vi "SVPO Integration (1 CH DBL WDT) with IC.vi"(6 "reset filters":bool, 7 "desired base units for length":i32(ring)=-1 items=["no change"=-1, "m"=0, "mm"=2, "microns"=3, "in"=1, "mils"=5], 8 "initial conditions":T1 {"filter state"."initial highpass filter state" format="%.2f"; "filter state"."initial integration fiter state"."y(n-2) state" format="%.2f"; "filter state"."initial integration fiter state"."x(n-2) state" format="%.2f"; "filter state"."initial integration fiter state"."y(n-1) state" format="%.2f"; "filter state"."initial integration fiter state"."x(n-1) state" format="%.2f"; "filter coefficents"."highpass filter coefficients"."Forward Coefficients" format="%.2f"; "filter coefficents"."highpass filter coefficients"."Reverse Coefficients" format="%.2f"; "filter coefficents"."integration filter coefficients"."alpha" format="%.2f"; "filter coefficents"."integration filter coefficients"."gamma" format="%.2f"; "filter coefficents"."integration filter coefficients"."beta" format="%.2f"}, 9 "highpass cutoff frequency [Hz]":dbl=1.0 format="%.2f", 11 "scaled signal [EU]":waveform(dbl)) -> (0 "final conditions":T1 {"filter state"."initial highpass filter state" format="%.2f"; "filter state"."initial integration fiter state"."y(n-2) state" format="%.2f"; "filter state"."initial integration fiter state"."x(n-2) state" format="%.2f"; "filter state"."initial integration fiter state"."y(n-1) state" format="%.2f"; "filter state"."initial integration fiter state"."x(n-1) state" format="%.2f"; "filter coefficents"."highpass filter coefficients"."Forward Coefficients" format="%.2f"; "filter coefficents"."highpass filter coefficients"."Reverse Coefficients" format="%.2f"; "filter coefficents"."integration filter coefficients"."alpha" format="%.2f"; "filter coefficents"."integration filter coefficients"."gamma" format="%.2f"; "filter coefficents"."integration filter coefficients"."beta" format="%.2f"}, 3 "integrated signal [EU*s]":waveform(dbl))   [LabVIEW 2017, in "SoundVib_Integration.lvlib"]
doc: "Converts acceleration to velocity or velocity to displacement using a time-domain waveform as the input. Wire data to the <B>scaled signal [EU]</B> input to determine the polymorphic instance to use or manually select the instance. This VI performs Single Integration only. You can pass the integrated signal [EU*s] output to the scaled signal [EU] input of second call to this VI to perform double integration."
uses:
  <vilib>/addons/Sound and Vibration/svt_Integration/SoundVib_Integration.lvlib
  <vilib>/addons/_NISVFA/_Shared subVIs/Controls/svc_Integration State.ctl
  <vilib>/addons/Sound and Vibration/svt_Integration/subVIs/svl_Apply Highpass Filter with IC.vi
  <vilib>/addons/Sound and Vibration/svt_Integration/subVIs/svl_Low Pass [Order 1] No State.vi
  <vilib>/addons/Sound and Vibration/svt_Integration/subVIs/svl_Design HighPass Filter.vi
  <vilib>/addons/Sound and Vibration/svt_Integration/subVIs/svl_RC Filter Coefficients.vi
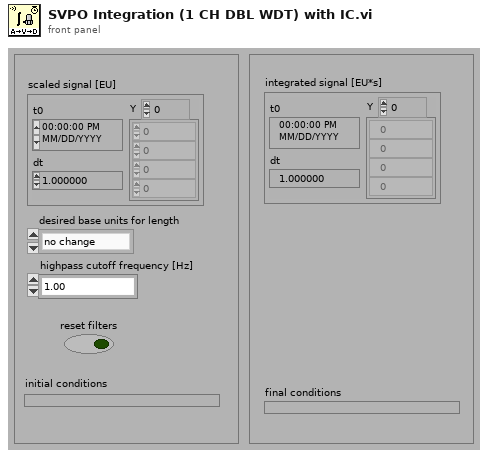
[diagram p1: front panel]
types:
  T1 = typedef "svc_Integration State.ctl" = cluster{"filter coefficents":cluster{"integration filter coefficients":cluster{"beta":dbl, "gamma":dbl, "alpha":dbl}, "highpass filter coefficients":cluster{"filter structure":enum32{"IIR 2nd Order", "IIR 4th Order"}, "Reverse Coefficients":dbl[], "Forward Coefficients":dbl[]}}, "filter state":cluster{"initial integration fiter state":cluster{"x(n-1) state":dbl, "y(n-1) state":dbl, "x(n-2) state":dbl, "y(n-2) state":dbl}, "initial highpass filter state":dbl[]}}
  T2 = enum16{"single integration", "double integration"}
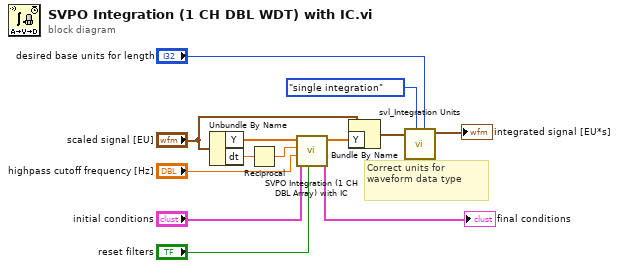
[diagram p0: block diagram]
diagram:
  # "Correct units for waveform data type"
  n1 = Unbundle By Name("scaled signal [EU]") -> ("Y"=w10:dbl[], "dt"=w12:dbl)
  n2 = Reciprocal(x=w12) -> (1/x=w11:dbl)
  n3 = call <vilib>:"SVPO Integration (1 CH DBL Array) with IC.vi"("reset filters"="reset filters", "initial conditions"="initial conditions", "highpass cutoff frequency [Hz]"="highpass cutoff frequency [Hz]", "sampling rate [Hz]"=w11, "scaled signal [EU]"=w10) -> ("final conditions"=→"final conditions":T1, "integrated signal [EU*s]"=w8:dbl[])  [unwired: 5 in]
  n4 = Bundle By Name(cluster="scaled signal [EU]", "Y"=w8) -> (w5:waveform(dbl))
  n5 = call <vilib>:"svl_Integration Units.vi"("desired base units for length"="desired base units for length", "integration type"=T2."single integration", "scaled signal [EU]"=w5) -> ("scaled signal out"=→"integrated signal [EU*s]":waveform(dbl))  [unwired: 6 in, 2 out]
